vi "LINC Get Connection Status.vi"(8 "error in (no error)":errorcluster, 11 "LINC session":refnum<class "LINC.lvclass">) -> (0 "error out":errorcluster, 2 "connected":bool[](array[boolean]), 3 "dup LINC session":refnum<class "LINC.lvclass">)   [LabVIEW 2018, in "STEPkgDriver_LINC.lvlib" / "LINC.lvclass"]
uses:
  LINC.lvclass
  LINC Global Session Mode.ctl
  STEPkgDriver_LINC.lvlib
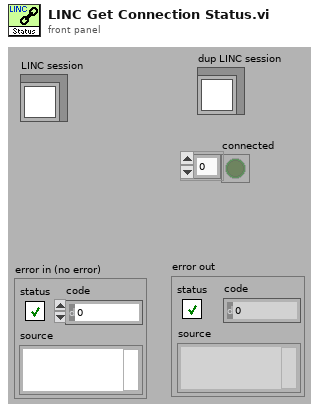
[diagram p1: front panel]
types:
  T1 = typedef "STEPkgDriver_LINC.lvlib/LINC Global Session Mode.ctl" = enum16{"INIT", "CLEAR", "ADD_SESSION", "SET_CONNECTION", "SET_LISTENER", "SET_REFERENCE", "GET_SESSION"}
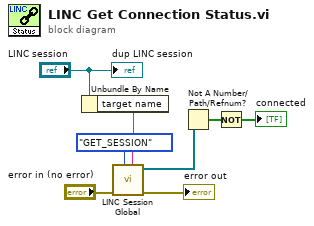
[diagram p0: block diagram]
diagram:
  n1 = Unbundle By Name("LINC session") -> ("target name"=w4:string)
  n2 = call "LINC Session Global.vi"("target name"=w4, "mode"=LINC_Global_Session_Mode."GET_SESSION", "error in (no error)"="error in (no error)") -> ("error out"=→"error out":errorcluster, "connections out"=w3:refnum<k5>[])  [unwired: 4 in, 3 out]
  n3 = Not A Number/Path/Refnum?(number/path/refnum=w3) -> (NaN/Path/Refnum?=w2:bool[])
  n4 = Not(x=w2) -> (.not. x?=→"connected":bool[])
  "dup LINC session" <- "LINC session"
